vi "test_harness_Hyst_op_fxp_16_5.vi"() -> ()   [LabVIEW 2017, in "Sat_Hyst_TestCase.lvclass"]
uses:
  Sat_Hyst_TestCase.lvclass
  C:/Program Files (x86)/National Instruments/LabVIEW 2017/vi.lib/addons/_JKI Toolkits/VI Tester/TestCase.llb/TestCase.lvclass
  <vilib>/rvi/DesktopExecutionNode/Execution/niFpgaDEN_Execute.vi
  <vilib>/rvi/DesktopExecutionNode/DesktopExecutionNode.xnode
  <userlib>/_VITAC/VITAC.lvlib
panel:
  out "y_out_mem":fxp<+/-,16,5>[](array[numeric])
  out "S_of_ik (expected)":sgl[](array[numeric])
  in  "error in (no error)":errorcluster
  out "error out":errorcluster
  out "TestCase out":refnum<class "Sat_Hyst_TestCase.lvclass">
  in  "TestCase in":refnum<class "Sat_Hyst_TestCase.lvclass">
  out "H_of_uk":fxp<+/-,32,10>[](array[numeric])
  out "sat(U) (expected, ML)":dbl[](array[numeric])
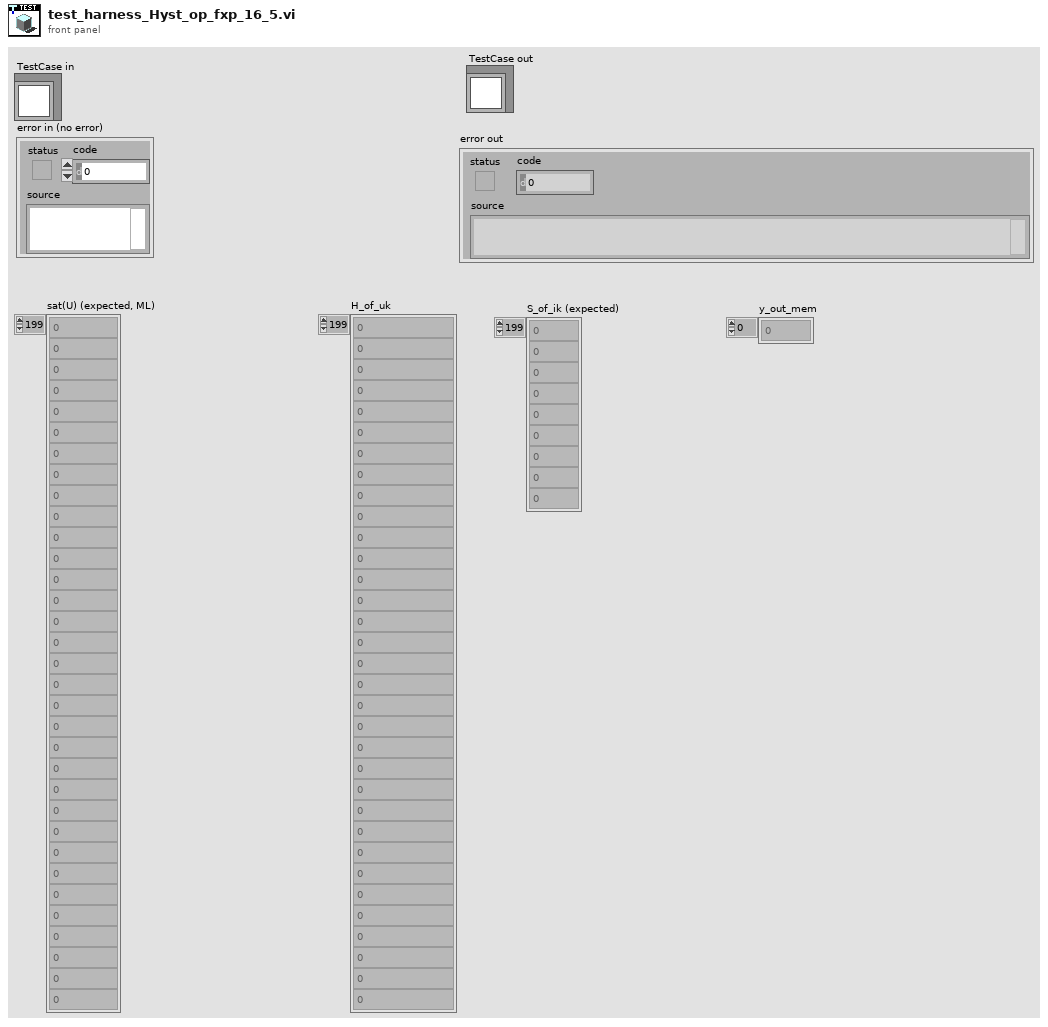
[diagram p1: front panel]
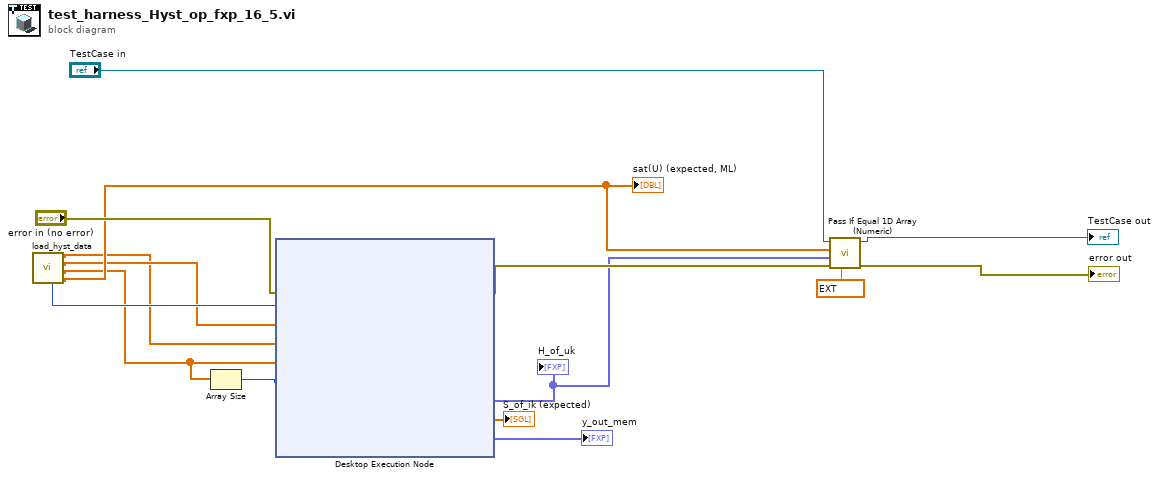
[diagram p0: block diagram]
diagram:
  n1 = call "load_hyst_data.vi"() -> ("Hyst(U_nom)"=w9:dbl[], "U_nom"=w5:dbl[], "wp"=w7:dbl[], "rps"=w6:dbl[], "N_sat"=w8:i32)  [unwired: 7 in]
  "sat(U) (expected, ML)" <- w9
  n2 = Array Size(array=w5) -> (size(s)=w4:i32)
  n3 = xnode "Desktop Execution Node"("Error In"="error in (no error)", "N_hyst"=w8, "w_s"=w7, "r_s"=w6, "uk"=w5, "numIter"=w4) -> ("Error Out"=w12:errorcluster, "H_of_uk"=w3:fxp<+/-,32,10>[], "S_of_ik (expected)"=→"S_of_ik (expected)":sgl[], "y_out_mem"=→"y_out_mem":fxp<+/-,16,5>[])
  "H_of_uk" <- w3
  n4 = call <userlib>:"Pass If Equal 1D Array (Numeric).vi"("delta (optional)"=ext 0.0001, "error in (no error)"=w12, "actual"=w3, "expected"=w9, "TestCase in"="TestCase in") -> ("error out"=→"error out":errorcluster, "TestCase out"=→"TestCase out":refnum<class "Sat_Hyst_TestCase.lvclass">)  [unwired: 5 in]
